vi "Global HCC Cluster ReadWrite.vi"(7 "Write?":bool, 8 "error in (no error)":errorcluster, 10 "configuration file path":path=path "D:/work/HCC_config.ini", 11 "Test Config In":T2={"Directories"={"Com Port Config Filename"=path "C:/Program Files/GE/Washer HCC/HCC_Com_Config.ini", "Save File Directory"=path "D:/Data", "Library Batch File"=path "c:/Program Files/GE/robocopy update.bat"}, "Test Information"={"Timeout"=1000, "Data Set ID"="HCC Rows A-C"}}) -> (0 "error out":errorcluster, 3 "Test Config Out":T2={"Directories"={"Com Port Config Filename"=path "D:/Work/HCC_Config.csv", "Save File Directory"=path "D:/Data", "Library Batch File"=path "c:/Data"}, "Test Information"={"Timeout"=1000, "Data Set ID"="HCC Rows A-D"}})   [LabVIEW 2011]
uses:
  HCC Global Cluster Type.ctl
  <vilib>/Utility/VariantDataType/Type.ctl
  <vilib>/Utility/config.llb/Write Key (Double).vi
  <vilib>/Utility/config.llb/Write Key (String).vi
  <vilib>/Utility/config.llb/Write Key (Path).vi
  <vilib>/Utility/config.llb/Write Key (I32).vi
  <vilib>/Utility/config.llb/Write Key (Boolean).vi
  <vilib>/Utility/config.llb/Read Key (String).vi
  <vilib>/Utility/config.llb/Read Key (Double).vi
  <vilib>/Utility/config.llb/Read Key (Path).vi
  <vilib>/Utility/config.llb/Read Key (I32).vi
  <vilib>/Utility/config.llb/Read Key (U32).vi
  <vilib>/Utility/config.llb/Read Key (Boolean).vi
  <vilib>/Utility/config.llb/NI_LVConfig.lvlib
  <vilib>/Utility/VariantDataType/VariantType.lvlib
panel:
  out "Type Enum":T1
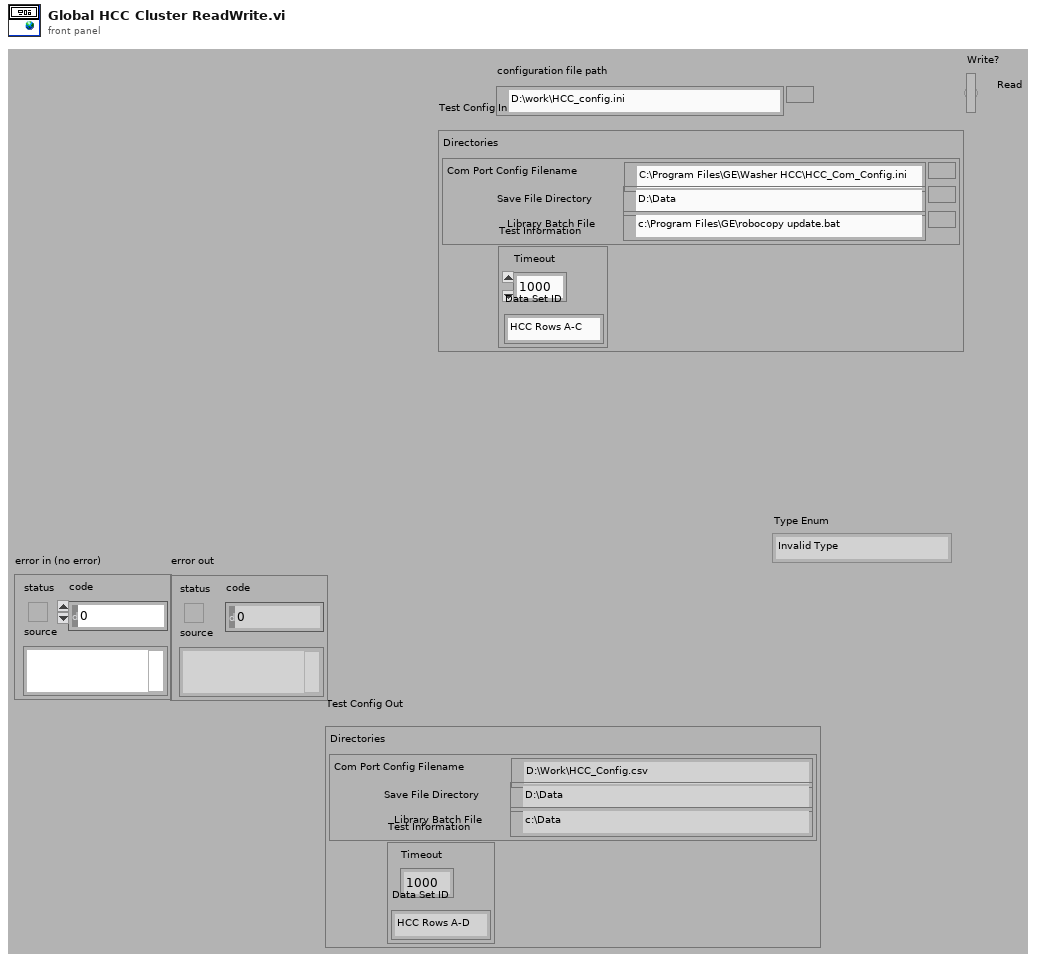
[diagram p1: front panel]
types:
  T1 = typedef "VariantType.lvlib/Type.ctl" = enum8{"Invalid Type", "Void", "I8", "I16", "I32", "I64", "U8", "U16", "U32", "U64", "Single Float", "Double Float", "Extended Float", "Single Complex", "Double Complex", "Extended Complex", "Enum U8", "Enum U16", "Enum U32", "Enum U64", "Single Float With Unit", "Double Float With Unit", "Extended Float With Unit", "Single Complex with Unit", "Double Complex with Unit", "Extended Complex with Unit", "Boolean", "String", "Path", "Picture", "Tag", "Array", "Cluster", "Variant", "LV Variant", "Waveform", "Timestamp", "Digital Waveform", "Digital Data", "ExpressData", "Refnum", "External Data", "VI", "Poly VI", "LabVIEW Class Instance", "Fixed Point"}
  T2 = typedef "HCC Global Cluster Type.ctl" = cluster{"Directories":cluster{"Com Port Config Filename":path, "Save File Directory":path, "Library Batch File":path}, "Test Information":cluster{"Timeout":i32, "Data Set ID":string}}
  T3 = typedef "NI_LVConfig.lvlib/Config Data RefNum.ctl" = refnum<k1>
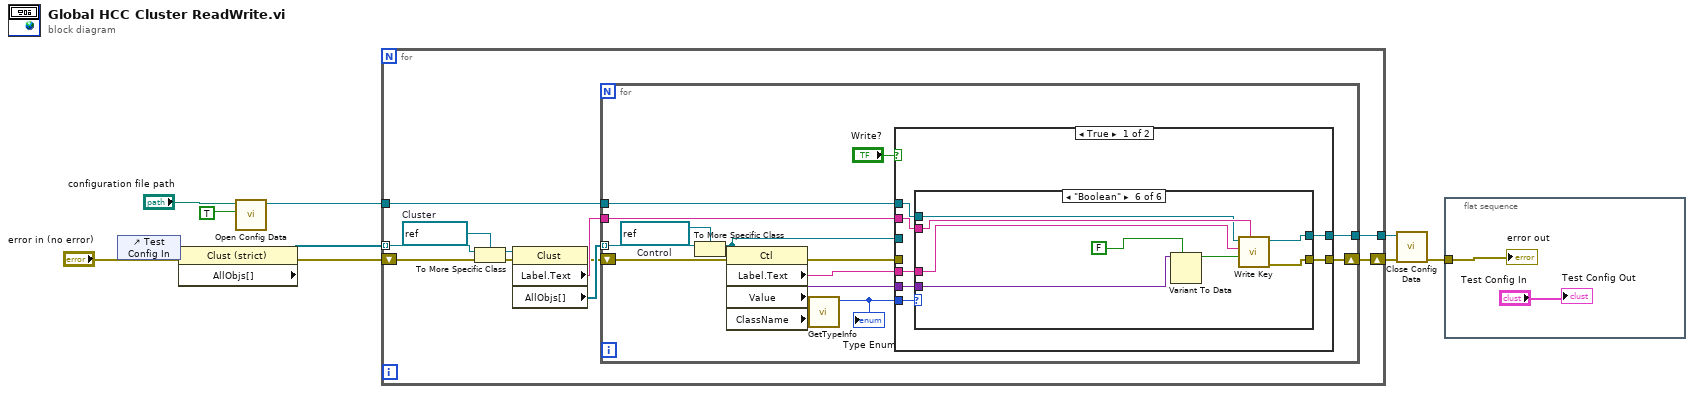
[diagram p0: block diagram]
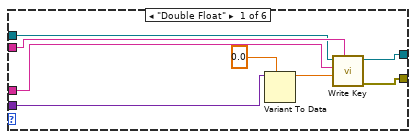
[diagram p2: hidden frame]
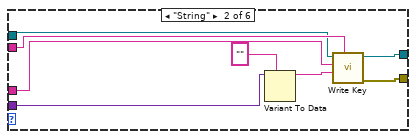
[diagram p3: hidden frame]
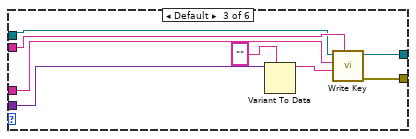
[diagram p4: hidden frame]
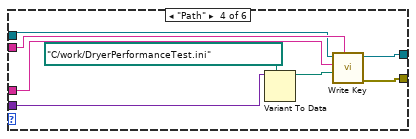
[diagram p5: hidden frame]
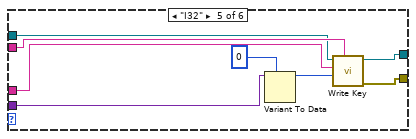
[diagram p6: hidden frame]
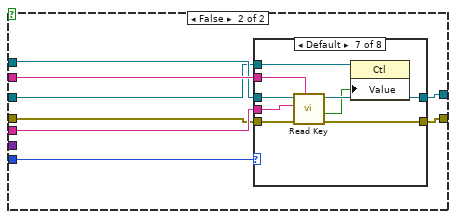
[diagram p7: hidden frame]
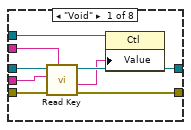
[diagram p8: hidden frame]
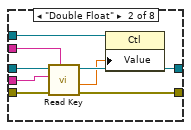
[diagram p9: hidden frame]
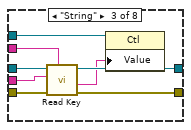
[diagram p10: hidden frame]
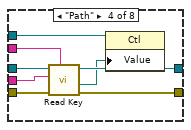
[diagram p11: hidden frame]
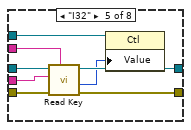
[diagram p12: hidden frame]
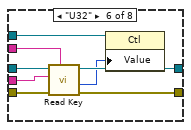
[diagram p13: hidden frame]
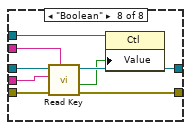
[diagram p14: hidden frame]
diagram:
  n1 = control-ref of="Test Config In"() -> (w10:refnum<vi>)
  n2 = property class="Clust (strict)"(reference=w10, error in="error in (no error)") -> (error out=w2:errorcluster, "AllObjs[]"=w9:refnum<vi>[])  [unwired: 1 out]
  n3 = call <vilib>:"Open Config Data.vi"("create file if necessary (T)"=TRUE, "configuration file path"="configuration file path") -> ("refnum"=w8:T3)  [unwired: 7 in, 2 out]
  n4 = for {
    tunnel: w9 -> [w21] mode=indexing
    tunnel: w8 -> [w16]
    tunnel: [w14] -> w6
    shift-right: [w15] -> w7
    shift-left: w2 -> [w13]
    w20 = refnum<vi> refnum  # Cluster
    n5 = To More Specific Class(target class=w20, reference=w21, error in=w13) -> (specific class reference=w19:refnum<vi>, error out=w12:errorcluster)
    n6 = property class="Clust"(reference=w19, error in=w12) -> (error out=w11:errorcluster, "Label.Text"=w17:string, "AllObjs[]"=w18:refnum<vi>[])  [unwired: 1 out]
    n7 = for {
      tunnel: w18 -> [w34] mode=indexing
      tunnel: w17 -> [w32]
      tunnel: w16 -> [w30]
      tunnel: [w28] -> w14
      shift-right: [w29] -> w15
      shift-left: w11 -> [w23]
      w33 = refnum<vi> refnum  # Control
      n8 = To More Specific Class(target class=w33, reference=w34) -> (specific class reference=w26:refnum<vi>)  [unwired: 1 in, 1 out]
      n9 = property class="Ctl" props=["Label", "Text", "Value", "ClassName"](reference=w26, error in=w23) -> (error out=w22:errorcluster, "Label.Text"=w31:string, "Value"=w24:variant)  [unwired: 2 out]
      n10 = call <vilib>:"GetTypeInfo.vi"("Variant"=w24) -> ("Type Enum"=w25:T1)  [unwired: 6 in, 4 out]
      "Type Enum" <- w25
      n11 = case shown="True" "Write?" {
        tunnel: w32 -> [w41 w97]
        tunnel: w31 -> [w40 w96]
        tunnel: w24 -> [w39 _]
        tunnel: w30 -> [w38 w95]
        tunnel: [w37 w94] -> w29
        tunnel: [w36 w93] -> w28
        tunnel: w26 -> [_ w92]
        tunnel: w25 -> [w35 w91]
        tunnel: w22 -> [_ w90]
        frame True {
          n12 = case shown="\"Boolean\"" w35 {
            tunnel: w41 -> [w49 w57 w65 w73 w81 w89]
            tunnel: w40 -> [w48 w56 w64 w72 w80 w88]
            tunnel: w39 -> [w47 w55 w63 w71 w79 w87]
            tunnel: w38 -> [w46 w54 w62 w70 w78 w86]
            tunnel: [w45 w53 w61 w69 w77 w85] -> w37
            tunnel: [w44 w52 w60 w68 w76 w84] -> w36
            frame "Double Float" {
              n13 = Variant To Data(type=0.0, Variant=w47) -> (data=w43:dbl)  [unwired: 1 in, 1 out]
              n14 = call-poly <vilib>:"Write Key.vi"("section"=w49, "value"=w43, "key"=w48, "refnum"=w46) -> ("error out"=w45:errorcluster, "refnum out"=w44:T3)  [unwired: 5 in, 1 out]
            }
            frame "String" {
              n15 = Variant To Data(type="" ("Label.Text"), Variant=w55) -> (data=w51:string)  [unwired: 1 in, 1 out]
              n16 = call-poly <vilib>:"Write Key.vi"("section"=w57, "value"=w51, "key"=w56, "refnum"=w54) -> ("error out"=w53:errorcluster, "refnum out"=w52:T3)  [unwired: 5 in, 1 out]
            }
            frame Default {
              n17 = Variant To Data(type="" ("Label.Text"), Variant=w63) -> (data=w59:string)  [unwired: 1 in, 1 out]
              n18 = call-poly <vilib>:"Write Key.vi"("section"=w65, "value"=w59, "key"=w64, "refnum"=w62) -> ("error out"=w61:errorcluster, "refnum out"=w60:T3)  [unwired: 5 in, 1 out]
            }
            frame "Path" {
              n19 = Variant To Data(type=path "C:/work/DryerPerformanceTest.ini" ("configuration file path 2"), Variant=w71) -> (data=w67:path)  [unwired: 1 in, 1 out]
              n20 = call-poly <vilib>:"Write Key.vi"("section"=w73, "value"=w67, "key"=w72, "refnum"=w70) -> ("error out"=w69:errorcluster, "refnum out"=w68:T3)  [unwired: 5 in, 1 out]
            }
            frame "I32" {
              n21 = Variant To Data(type=0, Variant=w79) -> (data=w75:i32)  [unwired: 1 in, 1 out]
              n22 = call-poly <vilib>:"Write Key.vi"("section"=w81, "value"=w75, "key"=w80, "refnum"=w78) -> ("error out"=w77:errorcluster, "refnum out"=w76:T3)  [unwired: 5 in, 1 out]
            }
            frame "Boolean" {
              n23 = Variant To Data(type=FALSE ("Write? 2"), Variant=w87) -> (data=w83:bool)  [unwired: 1 in, 1 out]
              n24 = call-poly <vilib>:"Write Key.vi"("section"=w89, "value"=w83, "key"=w88, "refnum"=w86) -> ("error out"=w85:errorcluster, "refnum out"=w84:T3)  [unwired: 5 in, 1 out]
            }
          }
        }
        frame False {
          n25 = case shown="Default" w91 {
            tunnel: w97 -> [w105 w113 w121 w122 w130 w138 w146 w154]
            tunnel: w96 -> [w104 w112 w120 w129 w137 w145 w153 w161]
            tunnel: w95 -> [w103 w111 w119 w128 w136 w144 w152 w160]
            tunnel: [w102 w110 w118 w127 w135 w143 w151 w159] -> w94
            tunnel: [w101 w109 w117 w126 w134 w142 w150 w158] -> w93
            tunnel: w92 -> [w99 w107 w115 w124 w132 w140 w148 w156]
            tunnel: w90 -> [w98 w106 w114 w123 w131 w139 w147 w155]
            frame "Void" {
              n26 = call-poly <vilib>:"Read Key.vi"("section"=w105, "error in (no error)"=w98, "key"=w104, "refnum"=w103) -> ("error out"=w102:errorcluster, "value"=w100:string, "refnum out"=w101:T3)  [unwired: 4 in, 1 out]
              n27 = property class="Ctl"(reference=w99, "Value"=w100) -> ()  [unwired: 1 in, 2 out]
            }
            frame "Double Float" {
              n28 = call-poly <vilib>:"Read Key.vi"("section"=w113, "error in (no error)"=w106, "key"=w112, "refnum"=w111) -> ("error out"=w110:errorcluster, "value"=w108:dbl, "refnum out"=w109:T3)  [unwired: 4 in, 1 out]
              n29 = property class="Ctl"(reference=w107, "Value"=w108) -> ()  [unwired: 1 in, 2 out]
            }
            frame "String" {
              n30 = call-poly <vilib>:"Read Key.vi"("section"=w121, "error in (no error)"=w114, "key"=w120, "refnum"=w119) -> ("error out"=w118:errorcluster, "value"=w116:string, "refnum out"=w117:T3)  [unwired: 4 in, 1 out]
              n31 = property class="Ctl"(reference=w115, "Value"=w116) -> ()  [unwired: 1 in, 2 out]
            }
            frame "Path" {
              n32 = call-poly <vilib>:"Read Key.vi"("section"=w122, "error in (no error)"=w123, "key"=w129, "refnum"=w128) -> ("error out"=w127:errorcluster, "value"=w125:path, "refnum out"=w126:T3)  [unwired: 4 in, 1 out]
              n33 = property class="Ctl"(reference=w124, "Value"=w125) -> ()  [unwired: 1 in, 2 out]
            }
            frame "I32" {
              n34 = call-poly <vilib>:"Read Key.vi"("section"=w130, "error in (no error)"=w131, "key"=w137, "refnum"=w136) -> ("error out"=w135:errorcluster, "value"=w133:i32, "refnum out"=w134:T3)  [unwired: 4 in, 1 out]
              n35 = property class="Ctl"(reference=w132, "Value"=w133) -> ()  [unwired: 1 in, 2 out]
            }
            frame "U32" {
              n36 = call-poly <vilib>:"Read Key.vi"("section"=w138, "error in (no error)"=w139, "key"=w145, "refnum"=w144) -> ("error out"=w143:errorcluster, "value"=w141:u32, "refnum out"=w142:T3)  [unwired: 4 in, 1 out]
              n37 = property class="Ctl"(reference=w140, "Value"=w141) -> ()  [unwired: 1 in, 2 out]
            }
            frame Default {
              n38 = call-poly <vilib>:"Read Key.vi"("section"=w146, "error in (no error)"=w147, "key"=w153, "refnum"=w152) -> ("error out"=w151:errorcluster, "value"=w149:bool, "refnum out"=w150:T3)  [unwired: 4 in, 1 out]
              n39 = property class="Ctl"(reference=w148, "Value"=w149) -> ()  [unwired: 1 in, 2 out]
            }
            frame "Boolean" {
              n40 = call-poly <vilib>:"Read Key.vi"("section"=w154, "error in (no error)"=w155, "key"=w161, "refnum"=w160) -> ("error out"=w159:errorcluster, "value"=w157:bool, "refnum out"=w158:T3)  [unwired: 4 in, 1 out]
              n41 = property class="Ctl"(reference=w156, "Value"=w157) -> ()  [unwired: 1 in, 2 out]
            }
          }
        }
      }
    }
  }
  n42 = call <vilib>:"Close Config Data.vi"("error in (no error)"=w7, "refnum"=w6) -> ("error out"=w1:errorcluster)  [unwired: 8 in, 1 out]
  n43 = flat-sequence {
    tunnel: w1 -> [w163]
    frame #0 {
      "Test Config Out" <- "Test Config In"
      "error out" <- w163
    }
  }
